vi "Read SN From mdata.ini.vi"(8 "错误输入（无错误）":errorcluster, 9 "用户事件":refnum<user-event>, 10 "isRead":refnum<vi>, 11 "String输入":refnum<vi>) -> (0 "错误输出":errorcluster)   [LabVIEW 2019]
uses:
  <vilib>/Utility/config.llb/Read Key (String).vi
  <vilib>/Utility/config.llb/NI_LVConfig.lvlib
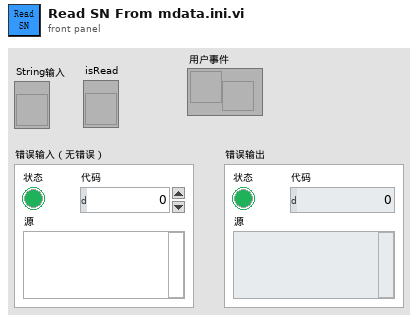
[diagram p1: front panel]
types:
  T1 = typedef "NI_LVConfig.lvlib/Config Data RefNum.ctl" = refnum<k1>
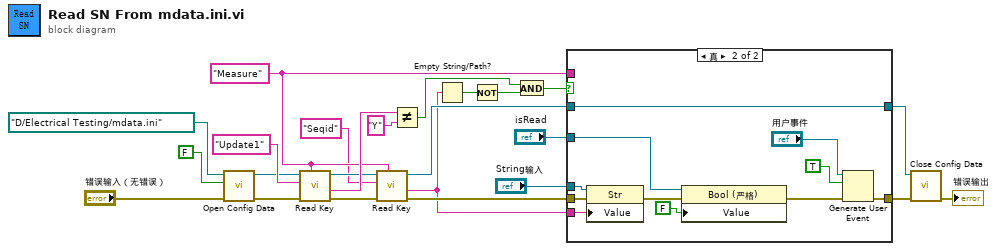
[diagram p0: block diagram]
diagram:
  w9 = "Measure" ("section")
  n1 = call <vilib>:"Open Config Data.vi"("error in (no error)"="错误输入（无错误）", "create file if necessary (T)"=FALSE, "configuration file path"=path "D:/Electrical Testing/mdata.ini") -> ("error out"=w17:errorcluster, "refnum"=w16:T1)  [unwired: 6 in, 1 out]
  n2 = call-poly <vilib>:"Read Key.vi"("section"=w9, "error in (no error)"=w17, "key"="Update1", "refnum"=w16) -> ("error out"=w13:errorcluster, "value"=w19:string, "refnum out"=w11:T1)  [unwired: 4 in, 1 out]
  n3 = call-poly <vilib>:"Read Key.vi"("section"=w9, "error in (no error)"=w13, "key"="Seqid", "refnum"=w11) -> ("error out"=w12:errorcluster, "value"=w3:string, "refnum out"=w10:T1)  [unwired: 4 in, 1 out]
  n4 = Not Equal?(x=w19, y="Y") -> (x != y?=w7:bool)
  n5 = Empty String/Path?(string/path=w3) -> (empty?=w6:bool)
  n6 = Not(x=w6) -> (.not. x?=w5:bool)
  n7 = And(x=w7, y=w5) -> (x .and. y?=w4:bool)
  n8 = case shown="真" w4 {
    tunnel: w10 -> [w26 w37]
    tunnel: w12 -> [w25 w36]
    tunnel: w9 -> [_ _]
    tunnel: "String输入" -> [_ w35]
    tunnel: [w26 w37] -> w22
    tunnel: [w25 w30] -> w23
    tunnel: "isRead" -> [_ w34]
    tunnel: w3 -> [_ w27]
    frame False {
    }
    frame True {
      n9 = property class="Str"(reference=w35, error in=w36, "Value"=w27) -> (error out=w33:errorcluster)  [unwired: 1 out]
      n10 = property class="Bool (严格)"(reference=w34, error in=w33, "Value"=FALSE ("值")) -> (error out=w31:errorcluster)  [unwired: 1 out]
      n11 = Generate User Event(user event="用户事件", event data cluster=TRUE, error in=w31) -> (error out=w30:errorcluster)  [unwired: 1 in, 1 out]
    }
  }
  n12 = call <vilib>:"Close Config Data.vi"("error in (no error)"=w23, "refnum"=w22) -> ("error out"=→"错误输出":errorcluster)  [unwired: 8 in, 1 out]
